vi "Run.vi"(8 "error in (no error)":errorcluster, 11 "User Interface in":refnum<class "User Interface.lvclass">) -> (0 "error out":errorcluster, 3 "User Interface out":refnum<class "User Interface.lvclass">)   [LabVIEW 2016, in "CLD Exam - ATM.lvlib" / "User Interface.lvclass"]
uses:
  User Interface.lvclass
  D:/Repos/Stream/software/Mediator/Classes/Mediated Actor/Mediated Actor.lvclass
  Mediator/Classes/Message Interface/Message Interface.lvclass
  User Interface.lvclass/User Interface.ctl
  Log/Application Log/Log Level.ctl
  Mediator/Classes/Message String/Message String.lvclass
  D:/Repos/Stream/software/Mediator/Classes/Message Interface/Message Interface.lvclass
  Mediator/Classes/Message Transport Queue/Message Transport Queue.lvclass
  D:/Repos/Stream/software/Mediator/Classes/Message Transport Interface/Message Transport Interface.lvclass
  Mediator/Classes/Mediated Actor/Mediated Actor.lvclass
  Log/Application Log/Application Log.lvclass
panel:
  in  "Enter":bool
  in  "User Input":string
  in  "Right Buttons":T1
  out "Right Menu":T2
  in  "Left Buttons":T1
  out "Left Menu":T2
  in  "Card Simulator":bool
  out "ATM Messages":string
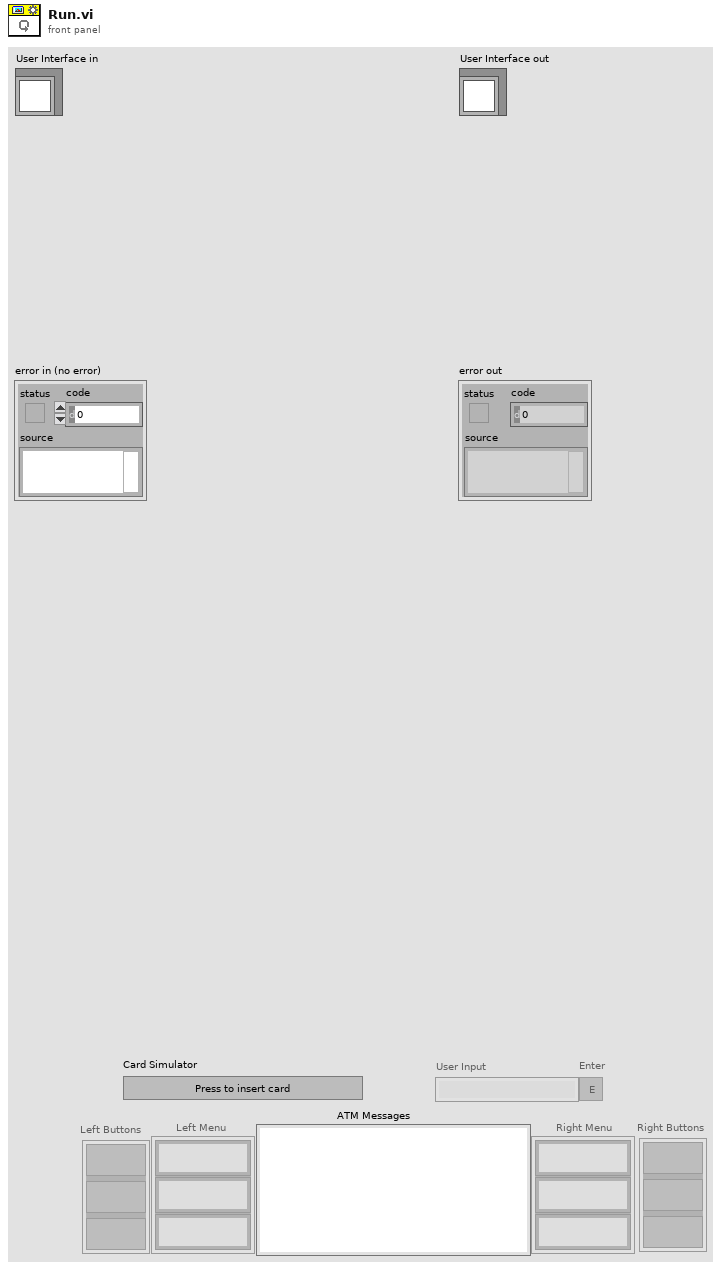
[diagram p1: front panel]
types:
  T1 = cluster{"Func Button":bool, "Func Button 2":bool, "Func Button 3":bool}
  T2 = cluster{"RFS String":string, "RFS String 2":string, "RFS String 3":string}
  T3 = cluster{"Main Message Updated":refnum<event-registration>, "Terminal Timed Out":refnum<event-registration>, "Card Inserted":refnum<event-registration>, "System Exit":refnum<event-registration>, "Account Action Completed":refnum<event-registration>, "Menu Updated":refnum<event-registration>, "To Self":refnum<event-registration>}
  T4 = typedef "Stream Log.lvlib/Application Log.lvclass/Log Level.ctl" = enum16{"Imperative", "Major", "Minor", "Debug", "Off"}
  T5 = enum8{"Enabled", "Disabled", "Disabled and Grayed Out"}
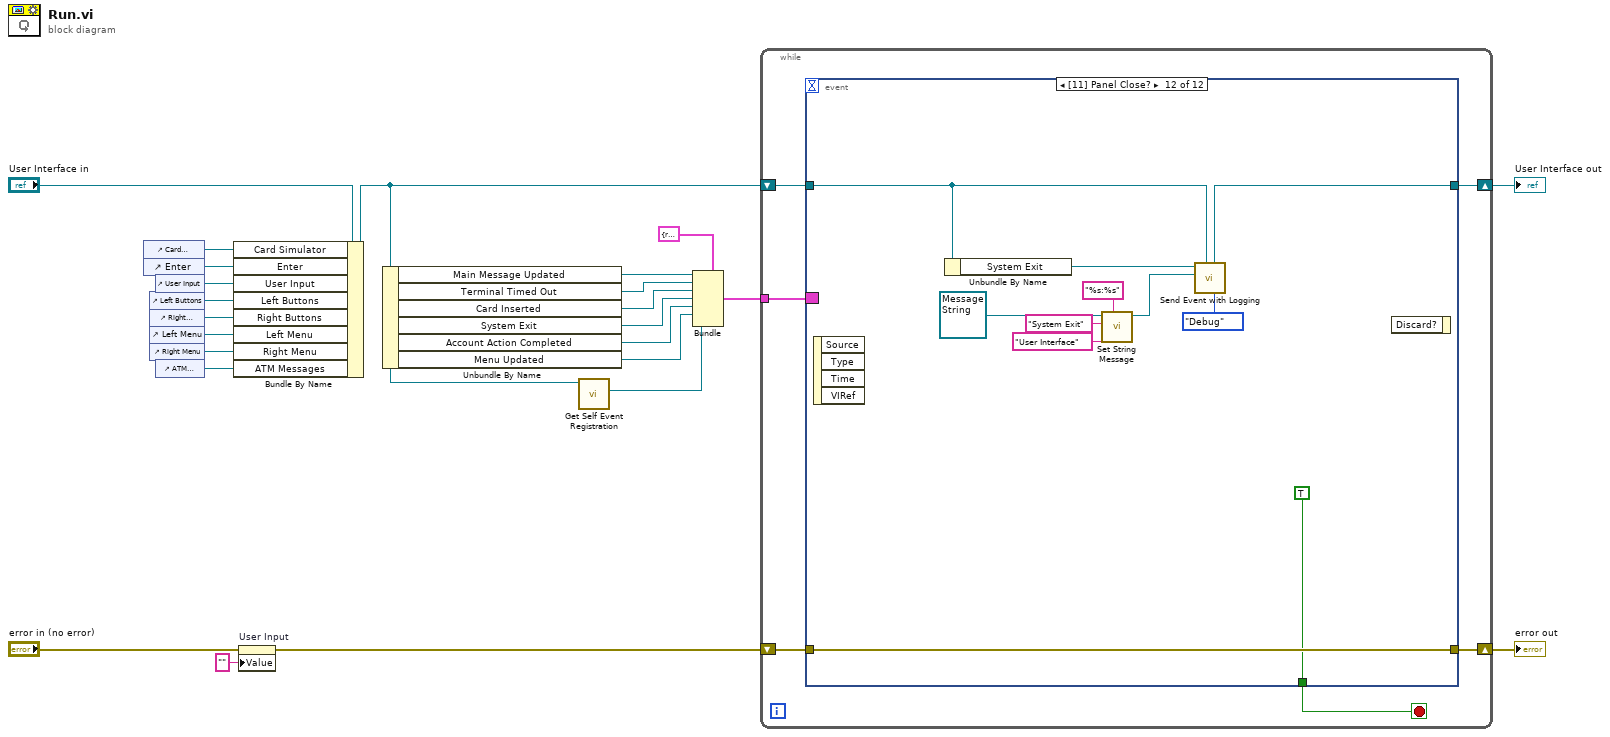
[diagram p0: block diagram]
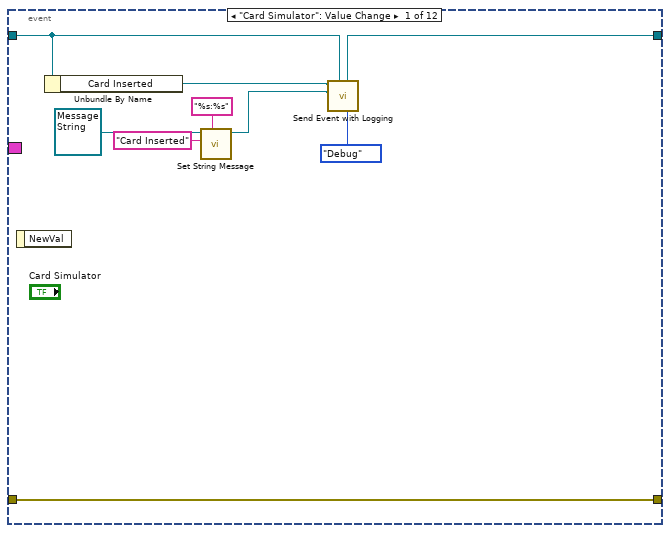
[diagram p2: hidden frame]
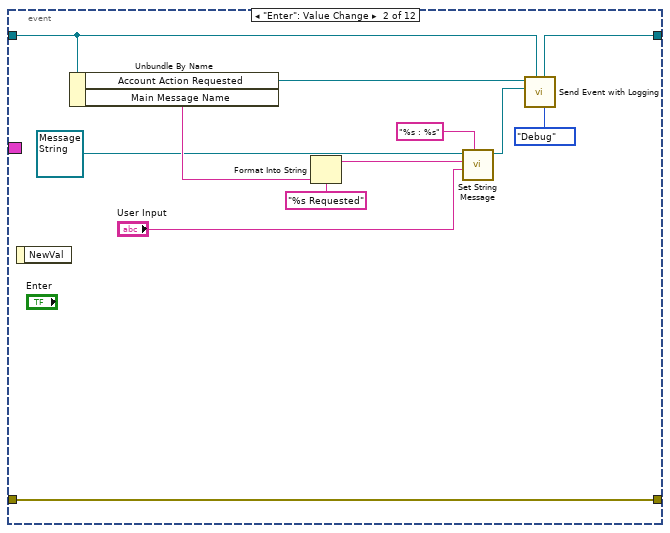
[diagram p3: hidden frame]
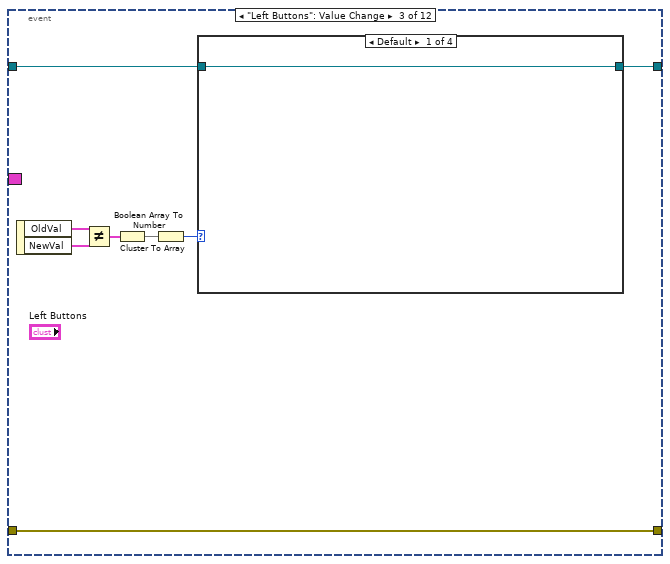
[diagram p4: hidden frame]
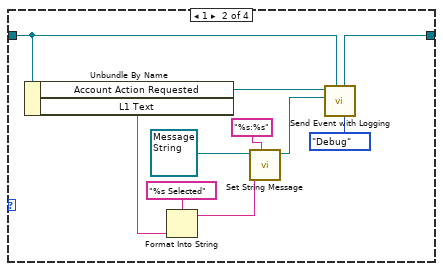
[diagram p5: hidden frame]
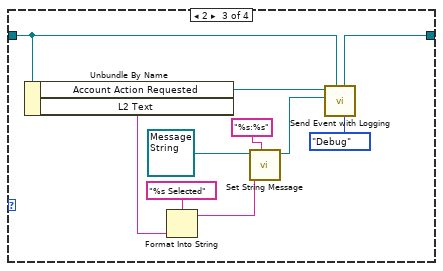
[diagram p6: hidden frame]
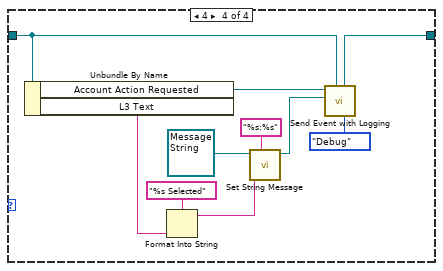
[diagram p7: hidden frame]
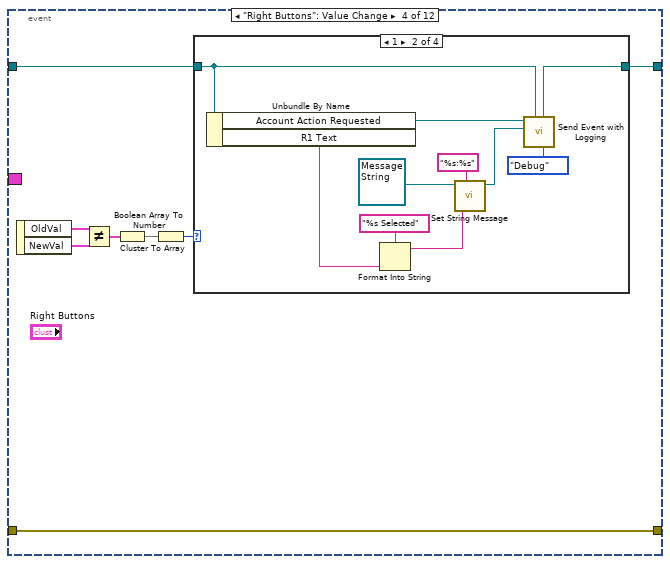
[diagram p8: hidden frame]
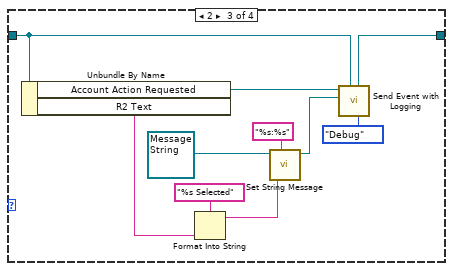
[diagram p10: hidden frame]
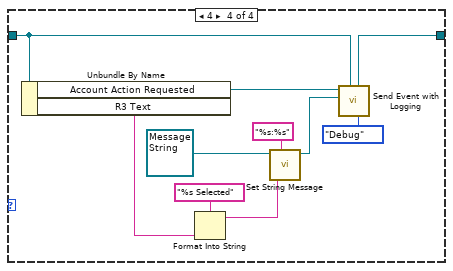
[diagram p11: hidden frame]
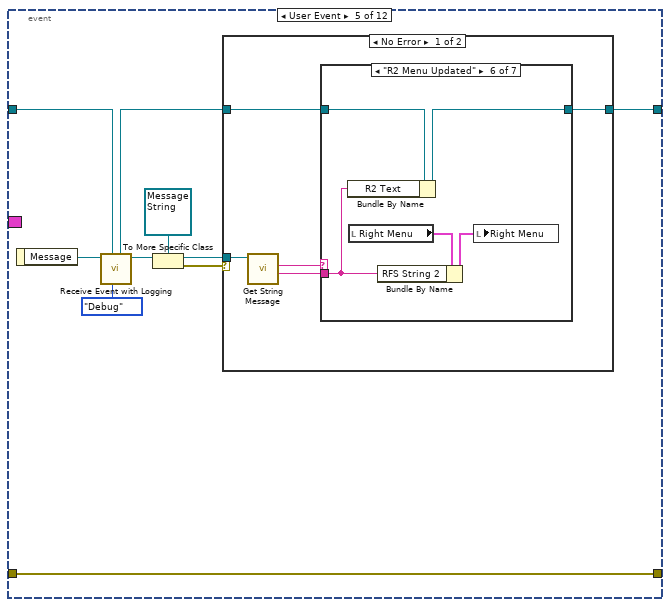
[diagram p12: hidden frame]
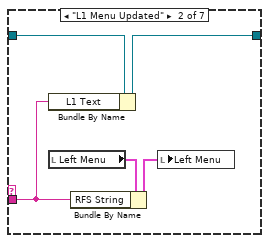
[diagram p14: hidden frame]
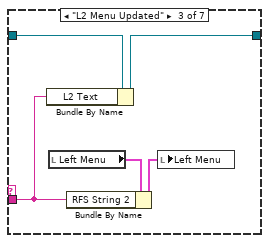
[diagram p15: hidden frame]
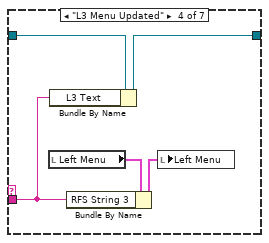
[diagram p16: hidden frame]
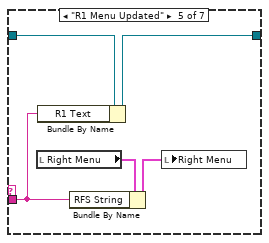
[diagram p17: hidden frame]
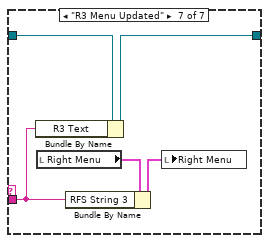
[diagram p18: hidden frame]
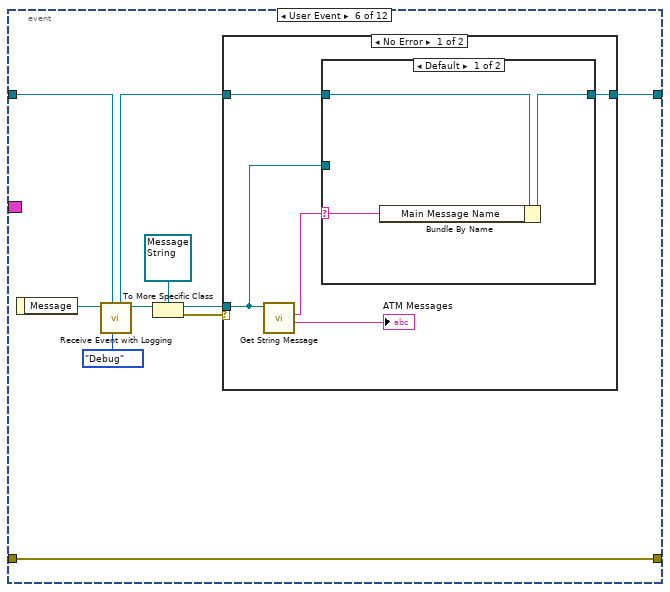
[diagram p20: hidden frame]
diagram:
  n1 = control-ref of="Card Simulator"() -> (w19:refnum<vi>)
  n2 = control-ref of="Enter"() -> (w18:refnum<vi>)
  n3 = control-ref of="Left Buttons"() -> (w16:refnum<vi>)
  n4 = control-ref of="Right Buttons"() -> (w15:refnum<vi>)
  n5 = control-ref of="Left Menu"() -> (w14:refnum<vi>)
  n6 = control-ref of="Right Menu"() -> (w13:refnum<vi>)
  n7 = control-ref of="User Input"() -> (w17:refnum<vi>)
  n8 = control-ref of="ATM Messages"() -> (w12:refnum<vi>)
  n9 = Bundle By Name(cluster="User Interface in", "Card Simulator"=w19, "Enter"=w18, "User Input"=w17, "Left Buttons"=w16, "Right Buttons"=w15, "Left Menu"=w14, "Right Menu"=w13, "ATM Messages"=w12) -> (w20:refnum<class "User Interface.lvclass">)
  n10 = property on="User Input" class="Str"(error in="error in (no error)", "Value"="" ("User Input")) -> (error out=w3:errorcluster)  [unwired: 1 in, 1 out]
  n11 = Unbundle By Name(w20) -> ("Main Message Updated"=w23:refnum<event-registration>, "Terminal Timed Out"=w22:refnum<event-registration>, "Card Inserted"=w10:refnum<event-registration>, "System Exit"=w9:refnum<event-registration>, "Account Action Completed"=w8:refnum<event-registration>, "Menu Updated"=w6:refnum<event-registration>)
  n12 = call "Get Self Event Registration.vi"("Mediated Actor in"=w20) -> ("Event Registration Refnum"=w5:refnum<event-registration>)  [unwired: 9 in, 1 out]
  n13 = Bundle(cluster=T3 {"Main Message Updated"=refnum, "Terminal Timed Out"=refnum, "Card Inserted"=refnum, "System Exit"=refnum, "Account Action Completed"=refnum, "Menu Updated"=refnum, "To Self"=refnum} ("output cluster"), "Main Message Updated"=w23, "Terminal Timed Out"=w22, "Card Inserted"=w10, "System Exit"=w9, "Account Action Completed"=w8, "Menu Updated"=w6, "To Self"=w5) -> (w7:T3)
  n14 = while {
    shift-right: [w29] -> w24
    shift-left: w20 -> [w30]
    tunnel: w7 -> [w28]
    shift-right: [w26] -> w11
    shift-left: w3 -> [w27]
    stop <- w25 stop-if-true
    n15 = event shown="[11] Panel Close?" {
      selector: w28 -> [_ _ _ _ _ _ _ _ _ _ _ _]
      dyn-events: _ -> [_ _ _ _ _ _ _ _ _ _ _ _]
      timeout: _ -> [_ _ _ _ _ _ _ _ _ _ _ _]
      tunnel: w30 -> [w33 w48 w59 w98 w134 w181 w208 w228 w247 w254 w273 w334]
      tunnel: [w32 w47 w56 w95 w131 w178 w212 w231 w246 w259 w277 w333] -> w29
      tunnel: w27 -> [w38 w50 w52 w91 w137 w184 w211 w234 w250 w260 w276 w340]
      tunnel: [w38 w50 w52 w91 w137 w184 w211 w234 w250 w260 w276 w340] -> w26
      tunnel: [_ _ _ _ _ _ _ _ TRUE _ _ TRUE] -> w25
      event "Card Simulator": Value Change {
        n16 = event-data() -> ()  [unwired: 1 in, 1 out]
        n17 = Unbundle By Name(w33) -> ("Card Inserted"=w36:refnum<class "Message Transport Queue.lvclass">)
        n18 = call "Set String Message.vi"("Format"="%s:%s", "Name"="Card Inserted", "Message String in"=refnum<class "Message String.lvclass"> refnum ("Stream Mediator.lvlib:Message String.lvclass")) -> ("Message String out"=w35:refnum<class "Message String.lvclass">)  [unwired: 7 in, 1 out]
        n19 = call "Send Event with Logging.vi"("Global Log Level"=Log_Level."Debug", "Mediated Actor in"=w33, "Message"=w35, "Message Transport Interface in"=w36) -> ("Mediated Actor out"=w32:refnum<class "User Interface.lvclass">)  [unwired: 6 in, 1 out]
      }
      event "Enter": Value Change {
        n20 = event-data() -> ()  [unwired: 1 in, 1 out]
        n21 = Unbundle By Name(w48) -> ("Account Action Requested"=w46:refnum<class "Message Transport Queue.lvclass">, "Main Message Name"=w42:string)
        n22 = Format Into String(format string="%s Requested", w42) -> (resulting string=w41:string)  [unwired: 2 in, 1 out]
        n23 = call "Set String Message.vi"("Format"="%s : %s", "Value"="User Input", "Name"=w41, "Message String in"=refnum<class "Message String.lvclass"> refnum ("Stream Mediator.lvlib:Message String.lvclass")) -> ("Message String out"=w45:refnum<class "Message String.lvclass">)  [unwired: 6 in, 1 out]
        n24 = call "Send Event with Logging.vi"("Global Log Level"=Log_Level."Debug", "Mediated Actor in"=w48, "Message"=w45, "Message Transport Interface in"=w46) -> ("Mediated Actor out"=w47:refnum<class "User Interface.lvclass">)  [unwired: 6 in, 1 out]
      }
      event "Left Buttons": Value Change {
        n25 = event-data() -> ("OldVal"=w58:T1, "NewVal"=w57:T1)  [unwired: 1 in]
        n26 = Not Equal?(x=w58, y=w57) -> (x != y?=w55:T1)
        n27 = Cluster To Array(cluster=w55) -> (array=w54:bool[])
        n28 = Boolean Array To Number(Boolean array=w54) -> (number=w53:u32)
        n29 = case shown="Default" w53 {
          tunnel: w59 -> [w60 w67 w77 w87]
          tunnel: [w60 w66 w76 w86] -> w56
          frame Default {
          }
          frame 1 {
            n30 = Unbundle By Name(w67) -> ("Account Action Requested"=w69:refnum<class "Message Transport Queue.lvclass">, "L1 Text"=w62:string)
            n31 = Format Into String(format string="%s Selected", w62) -> (resulting string=w63:string)  [unwired: 2 in, 1 out]
            n32 = call "Set String Message.vi"("Format"="%s:%s", "Name"=w63, "Message String in"=refnum<class "Message String.lvclass"> refnum ("Stream Mediator.lvlib:Message String.lvclass")) -> ("Message String out"=w68:refnum<class "Message String.lvclass">)  [unwired: 7 in, 1 out]
            n33 = call "Send Event with Logging.vi"("Global Log Level"=Log_Level."Debug", "Mediated Actor in"=w67, "Message"=w68, "Message Transport Interface in"=w69) -> ("Mediated Actor out"=w66:refnum<class "User Interface.lvclass">)  [unwired: 6 in, 1 out]
          }
          frame 2 {
            n34 = Unbundle By Name(w77) -> ("Account Action Requested"=w79:refnum<class "Message Transport Queue.lvclass">, "L2 Text"=w72:string)
            n35 = Format Into String(format string="%s Selected", w72) -> (resulting string=w73:string)  [unwired: 2 in, 1 out]
            n36 = call "Set String Message.vi"("Format"="%s:%s", "Name"=w73, "Message String in"=refnum<class "Message String.lvclass"> refnum ("Stream Mediator.lvlib:Message String.lvclass")) -> ("Message String out"=w78:refnum<class "Message String.lvclass">)  [unwired: 7 in, 1 out]
            n37 = call "Send Event with Logging.vi"("Global Log Level"=Log_Level."Debug", "Mediated Actor in"=w77, "Message"=w78, "Message Transport Interface in"=w79) -> ("Mediated Actor out"=w76:refnum<class "User Interface.lvclass">)  [unwired: 6 in, 1 out]
          }
          frame 4 {
            n38 = Unbundle By Name(w87) -> ("Account Action Requested"=w89:refnum<class "Message Transport Queue.lvclass">, "L3 Text"=w82:string)
            n39 = Format Into String(format string="%s Selected", w82) -> (resulting string=w83:string)  [unwired: 2 in, 1 out]
            n40 = call "Set String Message.vi"("Format"="%s:%s", "Name"=w83, "Message String in"=refnum<class "Message String.lvclass"> refnum ("Stream Mediator.lvlib:Message String.lvclass")) -> ("Message String out"=w88:refnum<class "Message String.lvclass">)  [unwired: 7 in, 1 out]
            n41 = call "Send Event with Logging.vi"("Global Log Level"=Log_Level."Debug", "Mediated Actor in"=w87, "Message"=w88, "Message Transport Interface in"=w89) -> ("Mediated Actor out"=w86:refnum<class "User Interface.lvclass">)  [unwired: 6 in, 1 out]
          }
        }
      }
      event "Right Buttons": Value Change {
        n42 = event-data() -> ("OldVal"=w97:T1, "NewVal"=w96:T1)  [unwired: 1 in]
        n43 = Not Equal?(x=w97, y=w96) -> (x != y?=w94:T1)
        n44 = Cluster To Array(cluster=w94) -> (array=w93:bool[])
        n45 = Boolean Array To Number(Boolean array=w93) -> (number=w92:u32)
        n46 = case shown="1" w92 {
          tunnel: w98 -> [w99 w108 w118 w128]
          tunnel: [w99 w107 w117 w127] -> w95
          frame Default {
          }
          frame 1 {
            n47 = Unbundle By Name(w108) -> ("Account Action Requested"=w106:refnum<class "Message Transport Queue.lvclass">, "R1 Text"=w101:string)
            n48 = Format Into String(format string="%s Selected", w101) -> (resulting string=w102:string)  [unwired: 2 in, 1 out]
            n49 = call "Set String Message.vi"("Format"="%s:%s", "Name"=w102, "Message String in"=refnum<class "Message String.lvclass"> refnum ("Stream Mediator.lvlib:Message String.lvclass")) -> ("Message String out"=w105:refnum<class "Message String.lvclass">)  [unwired: 7 in, 1 out]
            n50 = call "Send Event with Logging.vi"("Global Log Level"=Log_Level."Debug", "Mediated Actor in"=w108, "Message"=w105, "Message Transport Interface in"=w106) -> ("Mediated Actor out"=w107:refnum<class "User Interface.lvclass">)  [unwired: 6 in, 1 out]
          }
          frame 2 {
            n51 = Unbundle By Name(w118) -> ("Account Action Requested"=w116:refnum<class "Message Transport Queue.lvclass">, "R2 Text"=w111:string)
            n52 = Format Into String(format string="%s Selected", w111) -> (resulting string=w112:string)  [unwired: 2 in, 1 out]
            n53 = call "Set String Message.vi"("Format"="%s:%s", "Name"=w112, "Message String in"=refnum<class "Message String.lvclass"> refnum ("Stream Mediator.lvlib:Message String.lvclass")) -> ("Message String out"=w115:refnum<class "Message String.lvclass">)  [unwired: 7 in, 1 out]
            n54 = call "Send Event with Logging.vi"("Global Log Level"=Log_Level."Debug", "Mediated Actor in"=w118, "Message"=w115, "Message Transport Interface in"=w116) -> ("Mediated Actor out"=w117:refnum<class "User Interface.lvclass">)  [unwired: 6 in, 1 out]
          }
          frame 4 {
            n55 = Unbundle By Name(w128) -> ("Account Action Requested"=w126:refnum<class "Message Transport Queue.lvclass">, "R3 Text"=w121:string)
            n56 = Format Into String(format string="%s Selected", w121) -> (resulting string=w122:string)  [unwired: 2 in, 1 out]
            n57 = call "Set String Message.vi"("Format"="%s:%s", "Name"=w122, "Message String in"=refnum<class "Message String.lvclass"> refnum ("Stream Mediator.lvlib:Message String.lvclass")) -> ("Message String out"=w125:refnum<class "Message String.lvclass">)  [unwired: 7 in, 1 out]
            n58 = call "Send Event with Logging.vi"("Global Log Level"=Log_Level."Debug", "Mediated Actor in"=w128, "Message"=w125, "Message Transport Interface in"=w126) -> ("Mediated Actor out"=w127:refnum<class "User Interface.lvclass">)  [unwired: 6 in, 1 out]
          }
        }
      }
      event User Event {
        n59 = event-data() -> ("Message"=w136:refnum<class "Message Interface.lvclass">)  [unwired: 1 in]
        n60 = call "Receive Event with Logging.vi"("Global Log Level"=Log_Level."Debug", "Mediated Actor in"=w134, "Message"=w136) -> ("Message out"=w135:refnum<class "Message Interface.lvclass">, "Mediated Actor out"=w132:refnum<class "User Interface.lvclass">)  [unwired: 5 in, 2 out]
        n61 = To More Specific Class(target class=refnum<class "Message String.lvclass"> refnum ("Stream Mediator.lvlib:Message String.lvclass"), reference=w135) -> (specific class reference=w138:refnum<class "Message String.lvclass">, error out=w139:errorcluster)  [unwired: 1 in]
        n62 = case shown="No Error" w139 {
          tunnel: w138 -> [w144 _]
          tunnel: [w140 w176] -> w131
          tunnel: w132 -> [w141 w176]
          frame No Error {
            n63 = call "Get String Message.vi"("Message String in"=w144) -> ("Value"=w143:string, "Name"=w142:string)  [unwired: 7 in, 2 out]
            n64 = case shown="\"R2 Menu Updated\"" w142 {
              tunnel: w143 -> [_ w146 w151 w156 w161 w166 w171]
              tunnel: [w145 w147 w152 w157 w162 w167 w172] -> w140
              tunnel: w141 -> [w145 w148 w153 w158 w163 w168 w173]
              frame Default {
              }
              frame "L1 Menu Updated" {
                n65 = Bundle By Name(cluster=w148, "L1 Text"=w146) -> (w147:refnum<class "User Interface.lvclass">)
                n66 = local read "Left Menu"() -> (w150:T2)
                n67 = Bundle By Name(cluster=w150, "RFS String"=w146) -> (w149:T2)
                n68 = local write "Left Menu"(w149) -> ()
              }
              frame "L2 Menu Updated" {
                n69 = Bundle By Name(cluster=w153, "L2 Text"=w151) -> (w152:refnum<class "User Interface.lvclass">)
                n70 = local read "Left Menu"() -> (w155:T2)
                n71 = Bundle By Name(cluster=w155, "RFS String 2"=w151) -> (w154:T2)
                n72 = local write "Left Menu"(w154) -> ()
              }
              frame "L3 Menu Updated" {
                n73 = local read "Left Menu"() -> (w160:T2)
                n74 = Bundle By Name(cluster=w158, "L3 Text"=w156) -> (w157:refnum<class "User Interface.lvclass">)
                n75 = Bundle By Name(cluster=w160, "RFS String 3"=w156) -> (w159:T2)
                n76 = local write "Left Menu"(w159) -> ()
              }
              frame "R1 Menu Updated" {
                n77 = local read "Right Menu"() -> (w165:T2)
                n78 = Bundle By Name(cluster=w163, "R1 Text"=w161) -> (w162:refnum<class "User Interface.lvclass">)
                n79 = Bundle By Name(cluster=w165, "RFS String"=w161) -> (w164:T2)
                n80 = local write "Right Menu"(w164) -> ()
              }
              frame "R2 Menu Updated" {
                n81 = Bundle By Name(cluster=w168, "R2 Text"=w166) -> (w167:refnum<class "User Interface.lvclass">)
                n82 = local read "Right Menu"() -> (w170:T2)
                n83 = Bundle By Name(cluster=w170, "RFS String 2"=w166) -> (w169:T2)
                n84 = local write "Right Menu"(w169) -> ()
              }
              frame "R3 Menu Updated" {
                n85 = Bundle By Name(cluster=w173, "R3 Text"=w171) -> (w172:refnum<class "User Interface.lvclass">)
                n86 = local read "Right Menu"() -> (w175:T2)
                n87 = Bundle By Name(cluster=w175, "RFS String 3"=w171) -> (w174:T2)
                n88 = local write "Right Menu"(w174) -> ()
              }
            }
          }
          frame Error {
          }
        }
      }
      event User Event {
        n89 = event-data() -> ("Message"=w183:refnum<class "Message Interface.lvclass">)  [unwired: 1 in]
        n90 = call "Receive Event with Logging.vi"("Global Log Level"=Log_Level."Debug", "Mediated Actor in"=w181, "Message"=w183) -> ("Message out"=w182:refnum<class "Message Interface.lvclass">, "Mediated Actor out"=w179:refnum<class "User Interface.lvclass">)  [unwired: 5 in, 2 out]
        n91 = To More Specific Class(target class=refnum<class "Message String.lvclass"> refnum ("Stream Mediator.lvlib:Message String.lvclass"), reference=w182) -> (specific class reference=w185:refnum<class "Message String.lvclass">, error out=w186:errorcluster)  [unwired: 1 in]
        n92 = case shown="No Error" w186 {
          tunnel: w185 -> [w189 _]
          tunnel: w179 -> [w190 w204]
          tunnel: [w187 w204] -> w178
          frame No Error {
            n93 = call "Get String Message.vi"("Message String in"=w189) -> ("Value"=→"ATM Messages":string, "Name"=w188:string)  [unwired: 7 in, 2 out]
            n94 = case shown="Default" w188 {
              selector: w188 -> [w192 _]
              tunnel: w190 -> [w194 w197]
              tunnel: [w193 w196] -> w187
              tunnel: w189 -> [_ w195]
              frame Default {
                n95 = Bundle By Name(cluster=w194, "Main Message Name"=w192) -> (w193:refnum<class "User Interface.lvclass">)
              }
              frame "Terminate" {
                n96 = call "Get To Self Message Transport.vi"("Mediated Actor in"=w197) -> ("To Self"=w200:refnum<class "Message Transport Queue.lvclass">, "Mediated Actor out"=w202:refnum<class "User Interface.lvclass">)  [unwired: 9 in]
                n97 = call "Set String Message.vi"("Format"="%s:%s", "Name"="Terminate", "Message String in"=w195) -> ("Message String out"=w201:refnum<class "Message String.lvclass">)  [unwired: 7 in, 1 out]
                n98 = call "Send Event with Logging.vi"("Global Log Level"=Log_Level."Debug", "Mediated Actor in"=w202, "Message"=w201, "Message Transport Interface in"=w200) -> ("Mediated Actor out"=w196:refnum<class "User Interface.lvclass">)  [unwired: 6 in, 1 out]
              }
            }
          }
          frame Error {
          }
        }
      }
      event User Event {
        w205 = refnum<class "Message String.lvclass"> refnum ("Stream Mediator.lvlib:Message String.lvclass")
        n99 = event-data() -> ("Message"=w210:refnum<class "Message Interface.lvclass">)  [unwired: 1 in]
        n100 = call "Receive Event with Logging.vi"("Global Log Level"=Log_Level."Debug", "Mediated Actor in"=w208, "Message"=w210) -> ("Message out"=w209:refnum<class "Message Interface.lvclass">, "Mediated Actor out"=w207:refnum<class "User Interface.lvclass">)  [unwired: 5 in, 2 out]
        n101 = To More Specific Class(target class=w205, reference=w209) -> (specific class reference=w213:refnum<class "Message String.lvclass">, error out=w214:errorcluster)  [unwired: 1 in]
        n102 = case shown="No Error" w214 {
          tunnel: w213 -> [_ _]
          tunnel: [w216 w224] -> w212
          tunnel: w207 -> [w223 w224]
          tunnel: w205 -> [w221 _]
          frame No Error {
            n103 = call "Set String Message.vi"("Format"="%s:%s", "Name"="Initialize UI", "Message String in"=w221) -> ("Message String out"=w218:refnum<class "Message String.lvclass">)  [unwired: 7 in, 1 out]
            n104 = call "Get To Self Message Transport.vi"("Mediated Actor in"=w223) -> ("To Self"=w219:refnum<class "Message Transport Queue.lvclass">, "Mediated Actor out"=w217:refnum<class "User Interface.lvclass">)  [unwired: 9 in]
            n105 = call "Send Event with Logging.vi"("Global Log Level"=Log_Level."Debug", "Mediated Actor in"=w217, "Message"=w218, "Message Transport Interface in"=w219) -> ("Mediated Actor out"=w216:refnum<class "User Interface.lvclass">)  [unwired: 6 in, 1 out]
          }
          frame Error {
          }
        }
      }
      event User Event {
        w225 = refnum<class "Message String.lvclass"> refnum ("Stream Mediator.lvlib:Message String.lvclass")
        n106 = event-data() -> ("Message"=w230:refnum<class "Message Interface.lvclass">)  [unwired: 1 in]
        n107 = call "Receive Event with Logging.vi"("Global Log Level"=Log_Level."Debug", "Mediated Actor in"=w228, "Message"=w230) -> ("Message out"=w229:refnum<class "Message Interface.lvclass">, "Mediated Actor out"=w227:refnum<class "User Interface.lvclass">)  [unwired: 5 in, 2 out]
        n108 = To More Specific Class(target class=w225, reference=w229) -> (specific class reference=w232:refnum<class "Message String.lvclass">, error out=w233:errorcluster)  [unwired: 1 in]
        n109 = case shown="No Error" w233 {
          tunnel: w232 -> [_ _]
          tunnel: [w236 w244] -> w231
          tunnel: w227 -> [w243 w244]
          tunnel: w225 -> [w241 _]
          frame No Error {
            n110 = call "Set String Message.vi"("Format"="%s:%s", "Name"="Card Inserted", "Message String in"=w241) -> ("Message String out"=w238:refnum<class "Message String.lvclass">)  [unwired: 7 in, 1 out]
            n111 = call "Get To Self Message Transport.vi"("Mediated Actor in"=w243) -> ("To Self"=w239:refnum<class "Message Transport Queue.lvclass">, "Mediated Actor out"=w237:refnum<class "User Interface.lvclass">)  [unwired: 9 in]
            n112 = call "Send Event with Logging.vi"("Global Log Level"=Log_Level."Debug", "Mediated Actor in"=w237, "Message"=w238, "Message Transport Interface in"=w239) -> ("Mediated Actor out"=w236:refnum<class "User Interface.lvclass">)  [unwired: 6 in, 1 out]
          }
          frame Error {
          }
        }
      }
      event User Event {
        n113 = event-data() -> ("Message"=w248:refnum<class "Message Interface.lvclass">)  [unwired: 1 in]
        n114 = call "Receive Event with Logging.vi"("Global Log Level"=Log_Level."Debug", "Mediated Actor in"=w247, "Message"=w248) -> ("Mediated Actor out"=w246:refnum<class "User Interface.lvclass">)  [unwired: 5 in, 3 out]
      }
      event User Event {
        n115 = event-data() -> ("Message"=w256:refnum<class "Message Interface.lvclass">)  [unwired: 1 in]
        n116 = call "Receive Event with Logging.vi"("Global Log Level"=Log_Level."Debug", "Mediated Actor in"=w254, "Message"=w256) -> ("Message out"=w255:refnum<class "Message Interface.lvclass">, "Mediated Actor out"=w253:refnum<class "User Interface.lvclass">)  [unwired: 5 in, 2 out]
        n117 = To More Specific Class(target class=refnum<class "Message String.lvclass"> refnum ("Stream Mediator.lvlib:Message String.lvclass"), reference=w255) -> (specific class reference=w258:refnum<class "Message String.lvclass">)  [unwired: 1 in, 1 out]
        n118 = call "Get String Message.vi"("Message String in"=w258) -> ("Value"=w257:string)  [unwired: 7 in, 3 out]
        n119 = case shown="Default" w257 {
          tunnel: w253 -> [w261 w270]
          tunnel: [w261 w270] -> w259
          frame Default {
            n120 = Unbundle By Name(w261) -> ("Left Buttons"=w267:refnum<vi>, "Right Buttons"=w266:refnum<vi>, "Left Menu"=w265:refnum<vi>, "Right Menu"=w264:refnum<vi>)
            n121 = Build Array(w267, w266, w265, w264) -> (w263:refnum<vi>[])
            n122 = for {
              tunnel: w263 -> [w269] mode=indexing
              tunnel: T5."Enabled" ("Disabled") -> [w268]
              n123 = property class="Clust"(reference=w269, "DisabledEnum"=w268) -> ()  [unwired: 1 in, 2 out]
            }
          }
          frame "Failed" {
          }
        }
      }
      event User Event {
        n124 = event-data() -> ("Message"=w274:refnum<class "Message Interface.lvclass">)  [unwired: 1 in]
        n125 = call "Receive Event with Logging.vi"("Global Log Level"=Log_Level."Debug", "Mediated Actor in"=w273, "Message"=w274) -> ("Name"=w275:string, "Mediated Actor out"=w272:refnum<class "User Interface.lvclass">)  [unwired: 5 in, 2 out]
        n126 = case shown="\"Card Inserted\"" w275 {
          tunnel: [w278 w292 w296 w327] -> w277
          tunnel: w272 -> [w278 w292 w297 w327]
          frame Default {
          }
          frame "Initialize UI" {
            n127 = Unbundle By Name(w292) -> ("Card Simulator"=w283:refnum<vi>, "Enter"=w291:refnum<vi>, "User Input"=w290:refnum<vi>, "Left Buttons"=w289:refnum<vi>, "Right Buttons"=w288:refnum<vi>, "Left Menu"=w287:refnum<vi>, "Right Menu"=w286:refnum<vi>)
            n128 = Build Array(w291, w290, w289, w288, w287, w286) -> (w285:refnum<vi>[])
            n129 = for {
              tunnel: w285 -> [w294] mode=indexing
              tunnel: T5."Disabled and Grayed Out" ("Disabled") -> [w293]
              n130 = property class="Ctl"(reference=w294, "DisabledEnum"=w293) -> ()  [unwired: 1 in, 2 out]
            }
            n131 = property class="Bool (strict)"(reference=w283, "Value"=FALSE, "DisabledEnum"=T5."Enabled" ("Disabled")) -> ()  [unwired: 1 in, 2 out]
            "Left Menu" <- T2 {"RFS String"="", "RFS String 2"="", "RFS String 3"=""} ("Left Menu")
            "Right Menu" <- T2 {"RFS String"="", "RFS String 2"="", "RFS String 3"=""} ("Right Menu")
          }
          frame "Terminate" {
            n132 = Unbundle By Name(w297) -> ("System Exit"=w301:refnum<class "Message Transport Queue.lvclass">)
            n133 = Unbundle By Name(w297) -> ("Card Simulator"=w309:refnum<vi>, "Enter"=w316:refnum<vi>, "User Input"=w315:refnum<vi>, "Left Buttons"=w314:refnum<vi>, "Right Buttons"=w313:refnum<vi>, "Left Menu"=w312:refnum<vi>, "Right Menu"=w311:refnum<vi>)
            n134 = local write "Right Menu"(T2 {"RFS String"="", "RFS String 2"="", "RFS String 3"=""} ("Right Menu")) -> ()
            n135 = local write "Left Menu"(T2 {"RFS String"="", "RFS String 2"="", "RFS String 3"=""} ("Left Menu")) -> ()
            n136 = Build Array(w316, w315, w314, w313, w312, w311) -> (w310:refnum<vi>[])
            n137 = call "Set String Message.vi"("Format"="%s:%s", "Value"="User Interface", "Name"="System Exit", "Message String in"=refnum<class "Message String.lvclass"> refnum ("Stream Mediator.lvlib:Message String.lvclass")) -> ("Message String out"=w300:refnum<class "Message String.lvclass">)  [unwired: 6 in, 1 out]
            n138 = for {
              tunnel: w310 -> [w318] mode=indexing
              tunnel: T5."Disabled and Grayed Out" ("Disabled") -> [w317]
              n139 = property class="Ctl"(reference=w318, "DisabledEnum"=w317) -> ()  [unwired: 1 in, 2 out]
            }
            n140 = property class="Bool (strict)"(reference=w309, "Value"=FALSE, "DisabledEnum"=T5."Enabled" ("Disabled")) -> ()  [unwired: 1 in, 2 out]
            n141 = call "Send Event with Logging.vi"("Global Log Level"=Log_Level."Debug", "Mediated Actor in"=w297, "Message"=w300, "Message Transport Interface in"=w301) -> ("Mediated Actor out"=w296:refnum<class "User Interface.lvclass">)  [unwired: 6 in, 1 out]
          }
          frame "Card Inserted" {
            n142 = Unbundle By Name(w327) -> ("User Input"=w323:refnum<vi>, "Enter"=w326:refnum<vi>, "Card Simulator"=w321:refnum<vi>)
            n143 = Build Array(w323, w326) -> (w325:refnum<vi>[])
            n144 = for {
              tunnel: w325 -> [w329] mode=indexing
              tunnel: T5."Enabled" ("Disabled") -> [w328]
              n145 = property class="Ctl"(reference=w329, "DisabledEnum"=w328) -> ()  [unwired: 1 in, 2 out]
            }
            n146 = property class="Bool (strict)"(reference=w321, "DisabledEnum"=T5."Disabled and Grayed Out" ("Disabled")) -> ()  [unwired: 1 in, 2 out]
            n147 = property class="Str"(reference=w323, "Key Focus"=TRUE, "Value"="") -> ()  [unwired: 1 in, 2 out]
          }
        }
      }
      event Panel Close? {
        n148 = event-data() -> ()  [unwired: 1 in, 4 out]
        n149 = Unbundle By Name(w334) -> ("System Exit"=w336:refnum<class "Message Transport Queue.lvclass">)
        n150 = call "Set String Message.vi"("Format"="%s:%s", "Value"="User Interface", "Name"="System Exit", "Message String in"=refnum<class "Message String.lvclass"> refnum ("Stream Mediator.lvlib:Message String.lvclass")) -> ("Message String out"=w335:refnum<class "Message String.lvclass">)  [unwired: 6 in, 1 out]
        n151 = call "Send Event with Logging.vi"("Global Log Level"=Log_Level."Debug", "Mediated Actor in"=w334, "Message"=w335, "Message Transport Interface in"=w336) -> ("Mediated Actor out"=w333:refnum<class "User Interface.lvclass">)  [unwired: 6 in, 1 out]
        n152 = event-data() -> ()  [unwired: 2 in, 1 out]
      }
    }
  }
  "error out" <- w11
  "User Interface out" <- w24
